vi "Kinesis-get-motor-ID-v2.vi"() -> ()   [LabVIEW 2014]
doc: "André Romero - 2017\nandretec@ifsc.usp.br"
panel:
  in  "stop":bool
  out "GetPOS":dbl
  out "SerialNumber":u32
  out "Motor 1":bool
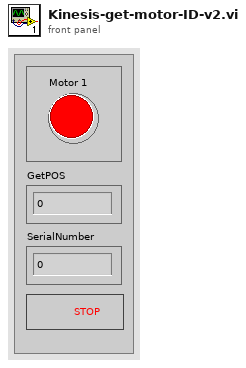
[diagram p1: front panel]
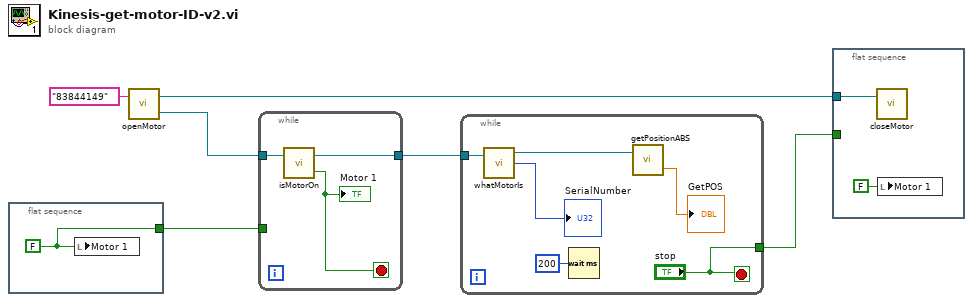
[diagram p0: block diagram]
diagram:
  n1 = flat-sequence {
    tunnel: [w7] -> w2
    frame #0 {
      w7 = FALSE ("Motor 1")
      n2 = local write "Motor 1"(w7) -> ()
    }
  }
  n3 = call "openMotor.vi"("S/N Motor"="83844149") -> ("Device"=w4:refnum<k24>, ".NET Refnum out"=w5:refnum<k24>)  [unwired: 1 in]
  n4 = while {
    tunnel: w4 -> [w10]
    tunnel: [w9] -> w6
    tunnel: w2 -> [_]
    stop <- w8 stop-if-true
    n5 = call "isMotorOn.vi"("Device"=w10) -> ("isConnected"=w8:bool, "Device out"=w9:refnum<k24>)  [unwired: 1 in]
    "Motor 1" <- w8
  }
  n6 = while {
    tunnel: w6 -> [w13]
    tunnel: ["stop"] -> w1
    stop <- "stop" stop-if-true
    n7 = call "whatMotorIs.vi"("Device in"=w13) -> ("SerialNumber"=→"SerialNumber":u32, "Device out"=w15:refnum<k24>)  [unwired: 3 in]
    n8 = Wait (ms)(milliseconds to wait=u32 200) -> ()  [unwired: 1 out]
    n9 = call "getPositionABS.vi"("Device"=w15) -> ("GetPOS"=→"GetPOS":dbl)  [unwired: 1 in, 1 out]
  }
  n10 = flat-sequence {
    tunnel: w5 -> [w18]
    tunnel: w1 -> [_]
    frame #0 {
      n11 = call "closeMotor.vi"(".NET Refnum in"=w18) -> ()  [unwired: 2 in]
      n12 = local write "Motor 1"(FALSE ("Motor 1")) -> ()
    }
  }
